vi "test_output_scale.vi"() -> ()   [LabVIEW 2018]
panel:
  in  "factor":u16
  out "Waveform Graph":i16[](graph)
  out "Array":bool[](array[boolean])
  in  "Data in":fxp<+/-,32,14>[](array[numeric])=[0.0, 0.0]
  out "Data out":fxp<+/-,16,14>[](array[numeric])
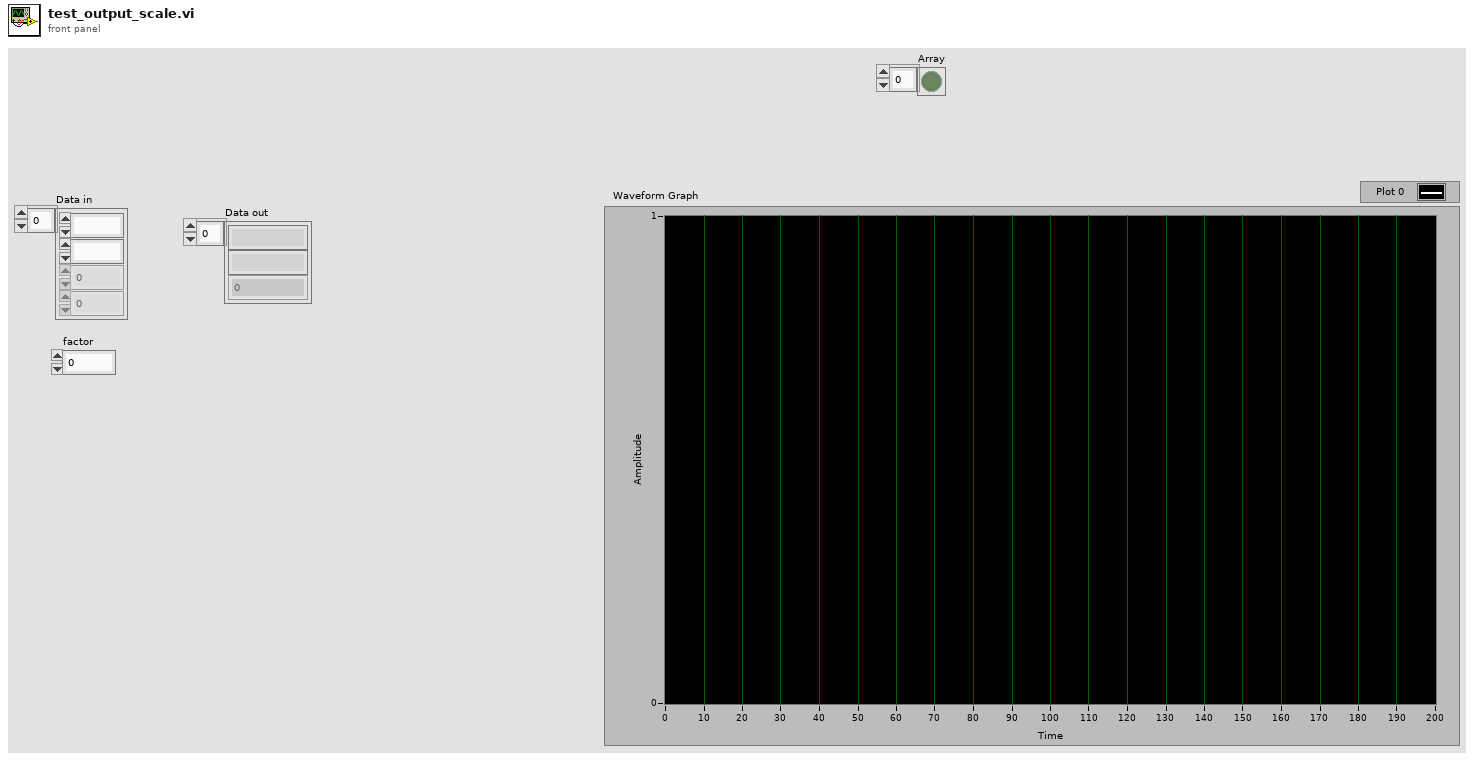
[diagram p1: front panel]
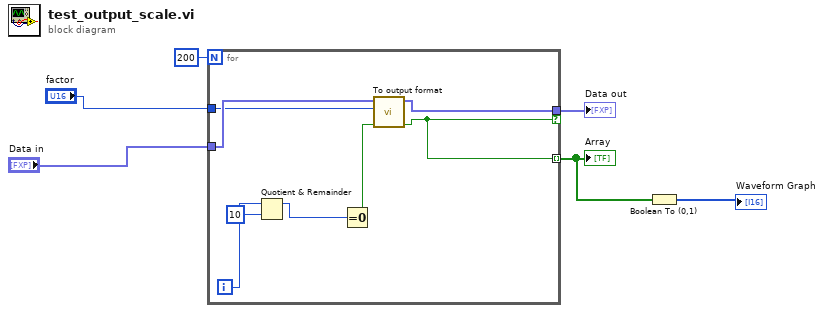
[diagram p0: block diagram]
diagram:
  n1 = for {
    N: 200 -> [_]
    tunnel: "Data in" -> [w11]
    tunnel: "factor" -> [w10]
    tunnel: [w9] -> w3 if=w7
    tunnel: [w7] -> w2 mode=indexing
    i -> [w14]
    n2 = Quotient & Remainder(x=w14, y=10) -> (x-y*floor(x/y)=w12:i32)  [unwired: 1 out]
    n3 = Equal To 0?(x=w12) -> (x = 0?=w8:bool)
    n4 = call "To output format.vi"("input valid"=w8, "factor"=w10, "Data in"=w11) -> ("output valid"=w7:bool, "Data out"=w9:fxp<+/-,16,14>[])  [unwired: 7 in]
  }
  "Data out" <- w3
  "Array" <- w2
  n5 = Boolean To (0,1)(Boolean=w2) -> (0, 1=→"Waveform Graph":i16[])
